vi "Actor Core.vi"(8 "error in":errorcluster, 11 "ImageHandler in":refnum<class "ImageHandler.lvclass">) -> (0 "error out":errorcluster, 3 "Actor out":refnum<class "Actor.lvclass">)   [LabVIEW 2022 SP3, in "ImageHandler.lvlib" / "ImageHandler.lvclass"]
doc: "(<B>Filename</B>: Actor Framework.lvlib:Actor.lvclass:Actor Core.vi)\n\nReceives messages to the actor, reacts to them, and initiates any error handling that may shut the actor down.\n\nDescendant classes may override this VI to append parallel tasks for the actor to complete while it handles messages. Overrides use the Call Parent Class Method node."
uses:
  ImageHandler.lvclass
  C:/Program Files/National Instruments/LabVIEW 2022/vi.lib/ActorFramework/Actor/Actor.lvclass
  <vilib>/ActorFramework/Actor/Actor.lvclass
  ImageHandler.lvclass/ImageHandler.ctl
  <vilib>/vision/Image Controls.llb/IMAQ Image.ctl
  <vilib>/ActorFramework/Actor/Actor.lvclass/Actor.ctl
  <vilib>/ActorFramework/Message Enqueuer/Message Enqueuer.lvclass/Message Enqueuer.ctl
  ImageHandler - Controller -- Interface/ImageHandler - Controller -- Interface Messages/Log Message Msg/Log Message Msg.lvclass/Log Message Msg.ctl
  ImageHandler Messages/Write Image Msg/Write Image Msg.lvclass/Write Image Msg.ctl
  <vilib>/ActorFramework/Message Enqueuer/Init from Existing Queue.vi
  <vilib>/ActorFramework/Message Enqueuer/Enqueue.vi
  ImageHandler - Controller -- Interface/ImageHandler - Controller -- Interface Messages/Log Message Msg/Log Message Msg.lvclass
  C:/Program Files/National Instruments/LabVIEW 2022/vi.lib/ActorFramework/Message/Message.lvclass
  ImageHandler Messages/Write Image Msg/Write Image Msg.lvclass
  <vilib>/ActorFramework/Message Priority Queue/Priority Enqueue.vi
  <vilib>/ActorFramework/Message Enqueuer/Message Enqueuer.lvclass
  BonTechDetector/BonTechDetector.lvlib
panel:
  out "time ms":u32
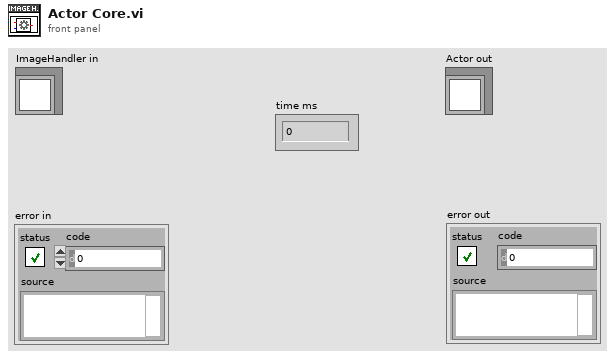
[diagram p1: front panel]
types:
  T1 = cluster{"Init":refnum<user-event>, "DeInit":refnum<user-event>, "Save":refnum<user-event>, "Stop":refnum<user-event>, "Display Mode":refnum<user-event>}
  T2 = cluster{"ImageWriteBuffer":u16[], "Image Width":i32, "Image Height":i32}
  T3 = typedef "IMAQ Image.ctl" = refnum<image>
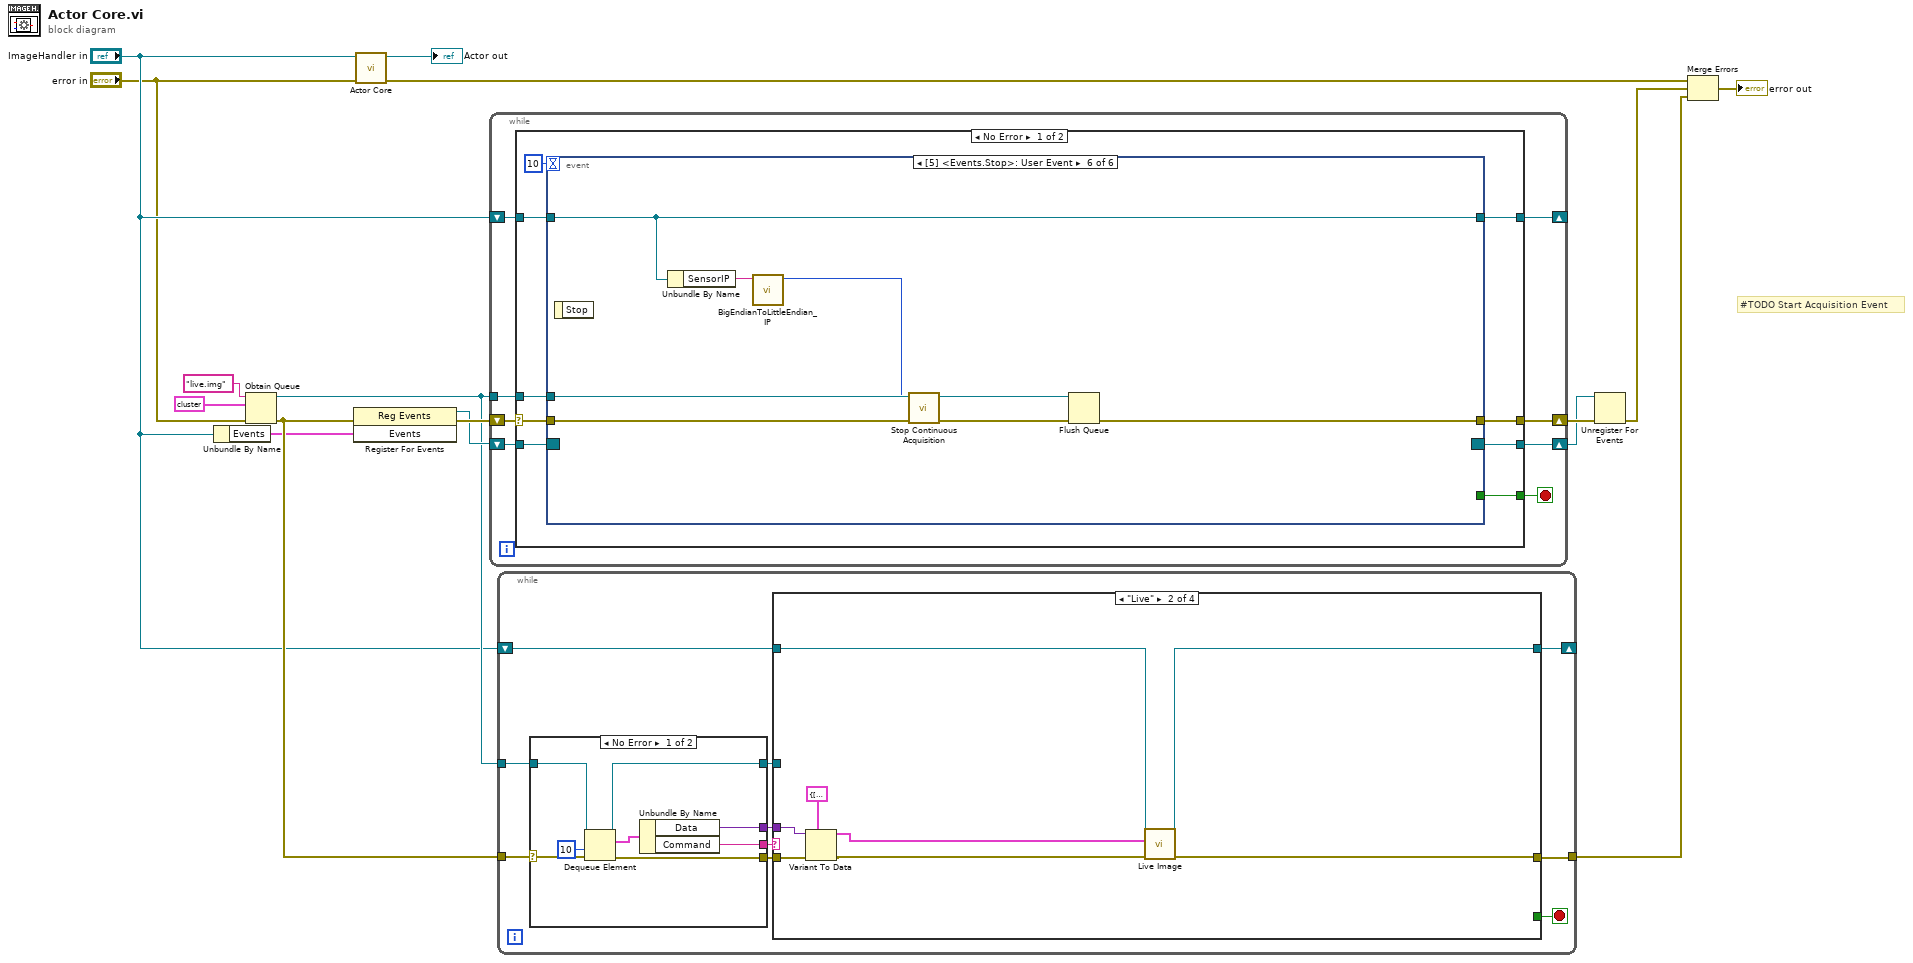
[diagram p0: block diagram]
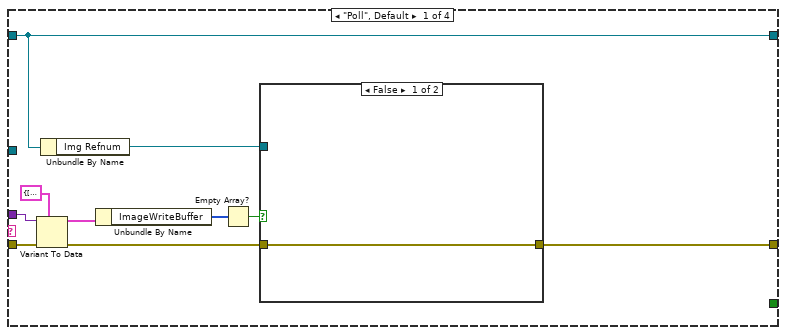
[diagram p2: hidden frame]
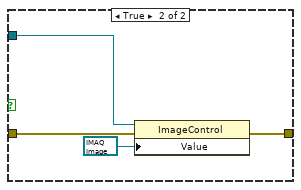
[diagram p3: hidden frame]
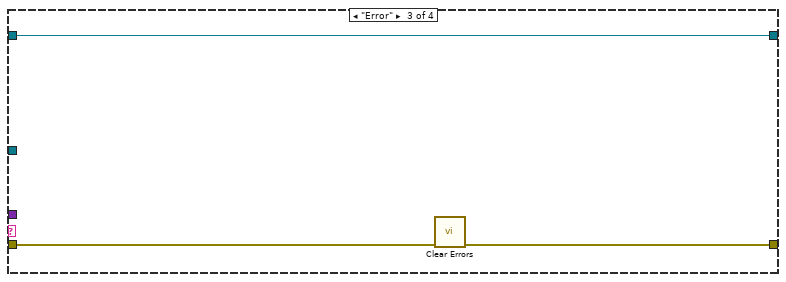
[diagram p4: hidden frame]
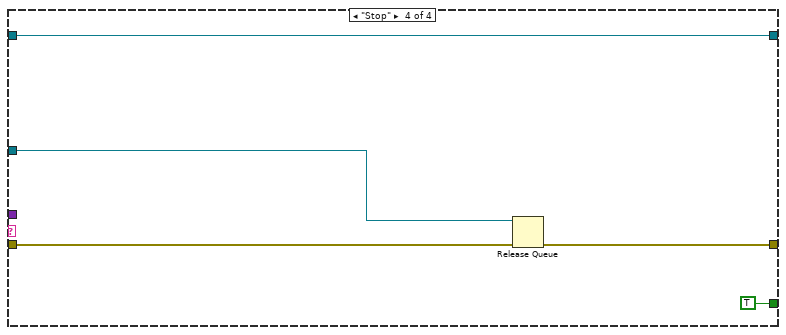
[diagram p5: hidden frame]
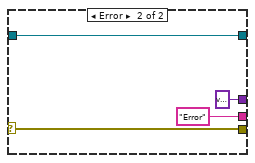
[diagram p6: hidden frame]
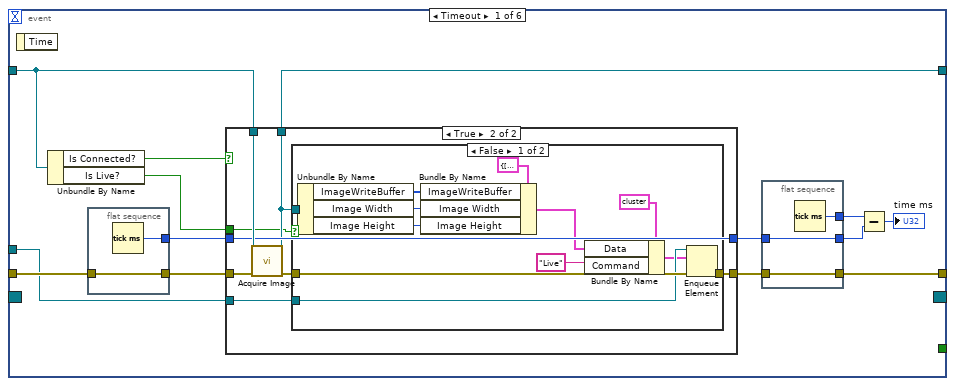
[diagram p7: hidden frame]
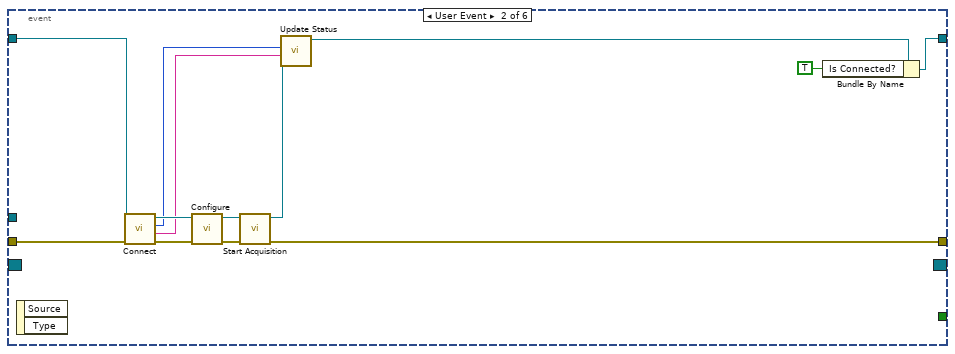
[diagram p10: hidden frame]
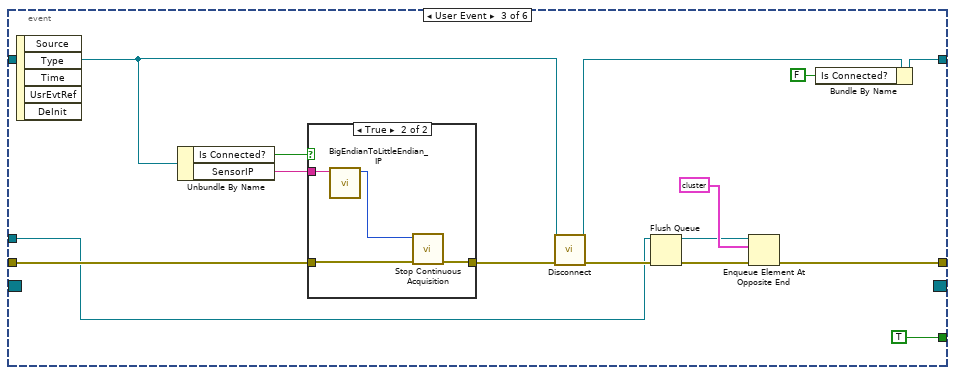
[diagram p11: hidden frame]
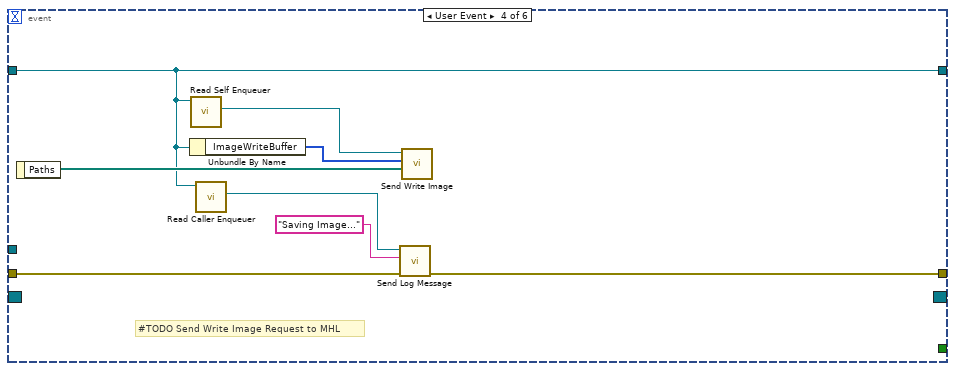
[diagram p13: hidden frame]
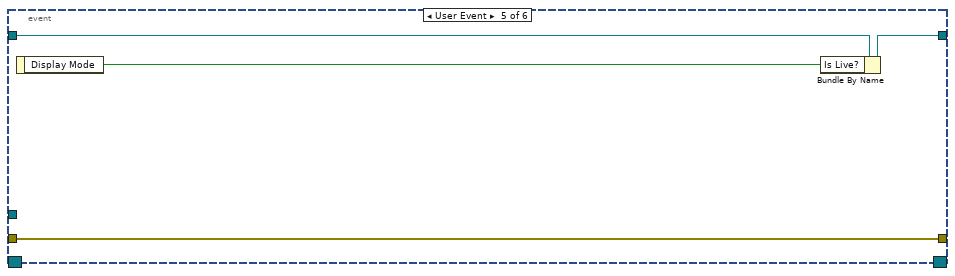
[diagram p14: hidden frame]
diagram:
  # "#TODO Start Acquisition Event"
  n1 = Unbundle By Name("ImageHandler in") -> ("Events"=w3:T1)
  n2 = Obtain Queue(name (unnamed)="live.img", element data type=cluster{"Data":variant, "Command":string} {"Data"=variant, "Command"=""}, error in (no error)="error in") -> (queue out=w6:refnum<queue>, error out=w5:errorcluster)  [unwired: 2 in, 1 out]
  n3 = register-events(error in=w5, w3) -> (reference out=w13:refnum<event-registration>, error out=w14:errorcluster)  [unwired: 1 in]
  n4 = call-parent "Actor Core.vi"("error in"="error in", "Actor in"="ImageHandler in") -> ("error out"=w16:errorcluster, "Actor out"=→"Actor out":refnum<class "Actor.lvclass">)  [unwired: 8 in]
  n5 = while {
    shift-right: [w23] -> _
    shift-left: "ImageHandler in" -> [w24]
    shift-right: [w22] -> w12
    shift-left: w14 -> [w19]
    shift-right: [w20] -> w11
    shift-left: w13 -> [w21]
    tunnel: w6 -> [w17]
    stop <- w18 stop-if-true
    n6 = case shown="No Error" w19 {
      selector: w19 -> [w27 w129]
      tunnel: w24 -> [w33 w130]
      tunnel: [w32 w130] -> w23
      tunnel: [w31 w129] -> w22
      tunnel: w21 -> [w30 w131]
      tunnel: [w28 w131] -> w20
      tunnel: [w25 _] -> w18
      tunnel: w17 -> [w26 _]
      frame No Error {
        n7 = event shown="[5] <Events.Stop>: User Event" {
          selector: w30 -> [_ _ _ _ _ _]
          dyn-events: [_ _ _ _ _ _] -> w28
          timeout: 10 -> [_ _ _ _ _ _]
          tunnel: w27 -> [w44 w89 w103 w111 w118 w127]
          tunnel: w33 -> [w46 w88 w93 w114 w121 w126]
          tunnel: [w47 w78 w101 w114 w120 w126] -> w32
          tunnel: [w40 w84 w96 w110 w118 w124] -> w31
          tunnel: w26 -> [w35 _ w91 _ _ w128]
          tunnel: [_ _ TRUE _ _ _] -> w25
          event Timeout {
            n8 = event-data() -> ()  [unwired: 1 in, 1 out]
            n9 = Unbundle By Name(w46) -> ("Is Connected?"=w45:bool, "Is Live?"=w34:bool)
            n10 = flat-sequence {
              tunnel: w44 -> [w75]
              tunnel: [w76] -> w43
              tunnel: [w75] -> w42
              frame #0 {
                n11 = Tick Count (ms)() -> (millisecond timer value=w76:u32)
              }
            }
            n12 = case shown="True" w45 {
              tunnel: w42 -> [w49 w58]
              tunnel: [w49 w54] -> w41
              tunnel: w46 -> [w50 w56]
              tunnel: [w50 w52] -> w47
              tunnel: w43 -> [w48 w55]
              tunnel: [w48 w55] -> w39
              tunnel: w35 -> [_ w53]
              tunnel: w34 -> [_ w51]
              frame False {
              }
              frame True {
                n13 = call "Acquire Image.vi"("error in (no error)"=w58, "ImageHandler in"=w56) -> ("error out"=w57:errorcluster, "ImageHandler out"=w52:refnum<class "ImageHandler.lvclass">)  [unwired: 8 in]
                n14 = case shown="False" w51 {
                  tunnel: w57 -> [w70 w71]
                  tunnel: [w69 w71] -> w54
                  tunnel: w53 -> [w68 _]
                  tunnel: w52 -> [w67 _]
                  frame False {
                    n15 = Unbundle By Name(w67) -> ("ImageWriteBuffer"=w65:u16[], "Image Width"=w63:i32, "Image Height"=w64:i32)
                    n16 = Bundle By Name(cluster=T2 {"ImageWriteBuffer"=[], "Image Width"=0, "Image Height"=0}, "ImageWriteBuffer"=w65, "Image Width"=w63, "Image Height"=w64) -> (w60:T2)
                    n17 = Bundle By Name(cluster=cluster{"Data":variant, "Command":string} {"Data"=variant, "Command"=""} ("element"), "Data"=w60, "Command"="Live") -> (w62:cluster{"Data":variant, "Command":string})
                    n18 = Enqueue Element(queue=w68, element=w62, error in (no error)=w70) -> (error out=w69:errorcluster)  [unwired: 1 in, 2 out]
                  }
                  frame True {
                  }
                }
              }
            }
            n19 = flat-sequence {
              tunnel: [w74] -> w38
              tunnel: w41 -> [w73]
              tunnel: [w73] -> w40
              tunnel: w39 -> [w72]
              tunnel: [w72] -> w37
              frame #0 {
                n20 = Tick Count (ms)() -> (millisecond timer value=w74:u32)
              }
            }
            n21 = Subtract(x=w38, y=w37) -> (x-y=→"time ms":u32)
          }
          event User Event {
            n22 = event-data() -> ()  [unwired: 1 in, 2 out]
            n23 = call "Connect.vi"("error in (no error)"=w89, "ImageHandler in"=w88) -> ("error out"=w86:errorcluster, "Serial Number"=w79:string, "Sensor Status"=w80:i32, "ImageHandler out"=w87:refnum<class "ImageHandler.lvclass">)  [unwired: 6 in]
            n24 = call "Configure.vi"("error in (no error)"=w86, "ImageHandler in"=w87) -> ("error out"=w85:errorcluster, "ImageHandler out"=w83:refnum<class "ImageHandler.lvclass">)  [unwired: 8 in]
            n25 = call "Start Acquisition.vi"("error in (no error)"=w85, "ImageHandler in"=w83) -> ("error out"=w84:errorcluster, "ImageHandler out"=w82:refnum<class "ImageHandler.lvclass">)  [unwired: 7 in, 1 out]
            n26 = call "Update Status.vi"("Serial Number"=w79, "Sensor Status"=w80, "ImageHandler in"=w82) -> ("ImageHandler out"=w81:refnum<class "ImageHandler.lvclass">)  [unwired: 7 in, 1 out]
            n27 = Bundle By Name(cluster=w81, "Is Connected?"=TRUE) -> (w78:refnum<class "ImageHandler.lvclass">)
          }
          event User Event {
            n28 = event-data() -> ()  [unwired: 1 in, 5 out]
            n29 = Unbundle By Name(w93) -> ("Is Connected?"=w99:bool, "SensorIP"=w94:string)
            n30 = case shown="True" w99 {
              tunnel: w103 -> [w105 w107]
              tunnel: [w105 w106] -> w102
              tunnel: w94 -> [_ w109]
              frame False {
              }
              frame True {
                n31 = call "BigEndianToLittleEndian_IP.vi"("IP String"=w109) -> ("IP Network Order"=w108:u32)  [unwired: 10 in]
                n32 = call "Stop Continuous Acquisition.vi"("error in (no error)"=w107, "nSensorIP"=w108) -> ("error out"=w106:errorcluster)  [unwired: 8 in, 1 out]
              }
            }
            n33 = call "Disconnect.vi"("error in (no error)"=w102, "ImageHandler in"=w93) -> ("error out"=w97:errorcluster, "ImageHandler out"=w104:refnum<class "ImageHandler.lvclass">)  [unwired: 8 in]
            n34 = Flush Queue(queue=w91, error in (no error)=w97) -> (queue out=w90:refnum<queue>, error out=w92:errorcluster)  [unwired: 1 out]
            n35 = Enqueue Element At Opposite End(queue=w90, element=cluster{"Data":variant, "Command":string} {"Data"=variant, "Command"="Stop"}, error in (no error)=w92) -> (error out=w96:errorcluster)  [unwired: 1 in, 2 out]
            n36 = Bundle By Name(cluster=w104, "Is Connected?"=FALSE) -> (w101:refnum<class "ImageHandler.lvclass">)
          }
          event User Event {
            # "#TODO Send Write Image Request to MHL"
            n37 = event-data() -> ("Paths"=w117:path[])  [unwired: 1 in]
            n38 = Unbundle By Name(w114) -> ("ImageWriteBuffer"=w116:u16[])
            n39 = call <vilib>:"Read Self Enqueuer.vi"("Actor"=w114) -> ("Self Enqueuer"=w115:refnum<class "Message Enqueuer.lvclass">)  [unwired: 10 in]
            n40 = call <vilib>:"Read Caller Enqueuer.vi"("Actor"=w114) -> ("Caller Enqueuer"=w113:refnum<class "Message Enqueuer.lvclass">)  [unwired: 10 in]
            n41 = call "Send Log Message.vi"("error in (no error)"=w111, "Log Message"="Saving Image...", "Message Enqueuer"=w113) -> ("error out"=w110:errorcluster)  [unwired: 7 in, 1 out]
            n42 = call "Send Write Image.vi"("Paths"=w117, "ImageWriteBuffer"=w116, "Message Enqueuer"=w115) -> ()  [unwired: 7 in, 2 out]
          }
          event User Event {
            n43 = event-data() -> ("Display Mode"=w119:bool)  [unwired: 1 in]
            n44 = Bundle By Name(cluster=w121, "Is Live?"=w119) -> (w120:refnum<class "ImageHandler.lvclass">)
          }
          event User Event {
            n45 = event-data() -> ()  [unwired: 1 in, 1 out]
            n46 = Unbundle By Name(w126) -> ("SensorIP"=w123:string)
            n47 = call "BigEndianToLittleEndian_IP.vi"("IP String"=w123) -> ("IP Network Order"=w122:u32)  [unwired: 10 in]
            n48 = call "Stop Continuous Acquisition.vi"("error in (no error)"=w127, "nSensorIP"=w122) -> ("error out"=w125:errorcluster)  [unwired: 8 in, 1 out]
            n49 = Flush Queue(queue=w128, error in (no error)=w125) -> (error out=w124:errorcluster)  [unwired: 2 out]
          }
        }
      }
      frame Error {
      }
    }
  }
  n50 = while {
    tunnel: w6 -> [w141]
    shift-right: [w133] -> _
    shift-left: "ImageHandler in" -> [w134]
    tunnel: w5 -> [w140]
    tunnel: [w136] -> w4
    stop <- w132 stop-if-true
    n51 = case shown="No Error" w140 {
      selector: w140 -> [w180 w182]
      tunnel: w141 -> [w178 w181]
      tunnel: [w174 "Error" ("Command")] -> w139
      tunnel: [w175 variant ("Data")] -> w138
      tunnel: [w179 w182] -> w137
      tunnel: [w177 w181] -> w135
      frame No Error {
        n52 = Dequeue Element(queue=w178, timeout in ms (-1)=10, error in (no error)=w180) -> (queue out=w177:refnum<queue>, element=w176:cluster{"Data":variant, "Command":string}, error out=w179:errorcluster)  [unwired: 1 out]
        n53 = Unbundle By Name(w176) -> ("Data"=w175:variant, "Command"=w174:string)
      }
      frame Error {
      }
    }
    n54 = case shown="\"Live\"" w139 {
      tunnel: w138 -> [w146 w163 _ _]
      tunnel: w137 -> [w151 w164 w165 w168]
      tunnel: [w150 w157 w166 w170] -> w136
      tunnel: w135 -> [_ _ _ w169]
      tunnel: w134 -> [w149 w160 w167 w172]
      tunnel: [w149 w159 w167 w172] -> w133
      tunnel: [_ _ _ TRUE] -> w132
      frame "Poll", Default {
        n55 = Variant To Data(error in=w151, type=T2 {"ImageWriteBuffer"=[], "Image Width"=0, "Image Height"=0}, Variant=w146) -> (data=w144:T2, error out=w147:errorcluster)
        n56 = Unbundle By Name(w149) -> ("Img Refnum"=w148:refnum<vi>)
        n57 = Unbundle By Name(w144) -> ("ImageWriteBuffer"=w143:u16[])
        n58 = Empty Array?(array=w143) -> (empty?=w142:bool)
        n59 = case shown="False" w142 {
          tunnel: w147 -> [w152 w156]
          tunnel: [w152 w155] -> w150
          tunnel: w148 -> [_ w154]
          frame False {
          }
          frame True {
            n60 = property class="ImageControl"(reference=w154, error in=w156, "Value"=T3 refnum ("ImaqLiveBuffer")) -> (error out=w155:errorcluster)  [unwired: 1 out]
          }
        }
      }
      frame "Live" {
        n61 = Variant To Data(error in=w164, type=T2 {"ImageWriteBuffer"=[], "Image Width"=0, "Image Height"=0}, Variant=w163) -> (data=w161:T2, error out=w162:errorcluster)
        n62 = call "Live Image.vi"("error in (no error)"=w162, "Live.Data"=w161, "ImageHandler in"=w160) -> ("error out"=w157:errorcluster, "ImageHandler out"=w159:refnum<class "ImageHandler.lvclass">)  [unwired: 7 in]
      }
      frame "Error" {
        n63 = call <vilib>:"Clear Errors.vi"("error in (no error)"=w165) -> ("error out"=w166:errorcluster)  [unwired: 5 in, 1 out]
      }
      frame "Stop" {
        n64 = Release Queue(queue=w169, error in (no error)=w168) -> (error out=w170:errorcluster)  [unwired: 1 in, 2 out]
      }
    }
  }
  n65 = Unregister For Events(event registration refnum=w11, error in=w12) -> (error out=w7:errorcluster)
  n66 = Merge Errors(w16, w7, w4) -> (→"error out":errorcluster)
